vi "Save Selected Area in Image.vi"(6 "Selected Area in Object":T3, 7 "Saved Image File Format":T1, 8 "error in (no error)":errorcluster, 10 "Image Data":T2, 11 "File Path in":path) -> (0 "error out":errorcluster, 3 "File Path out":path)   [LabVIEW 2021]
uses:
  Selected Area in Object.ctl
  <vilib>/picture/picture.llb/imagedata.ctl
  Pictures/Save File Format.ctl
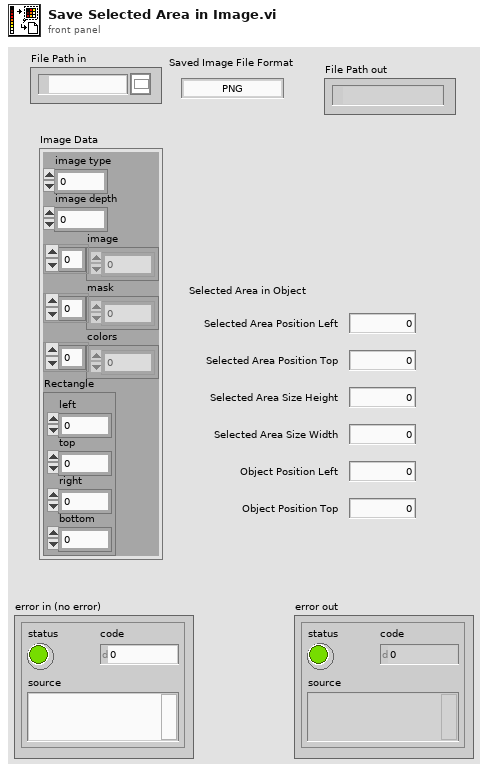
[diagram p1: front panel]
types:
  T1 = typedef "Save File Format.ctl" = enum16{"PNG", "JPEG", "BMP"}
  T2 = typedef "imagedata.ctl" = cluster{"image type":i32, "image depth":i32, "image":u8[], "mask":u8[], "colors":u32[], "Rectangle":cluster{"left":i16, "top":i16, "right":i16, "bottom":i16}}
  T3 = typedef "Selected Area in Object.ctl" = cluster{"Selected Area Position Left":i32, "Selected Area Position Top":i32, "Selected Area Size Height":u32, "Selected Area Size Width":u32, "Object Position Left":i32, "Object Position Top":i32}
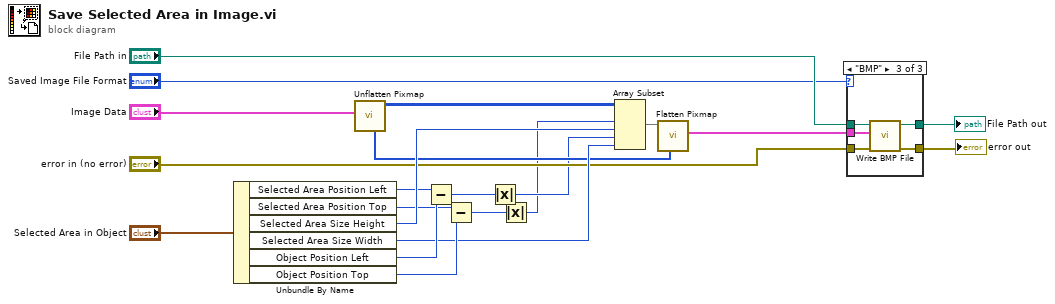
[diagram p0: block diagram]
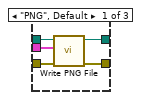
[diagram p2: hidden frame]
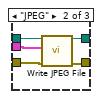
[diagram p3: hidden frame]
diagram:
  n1 = Unbundle By Name("Selected Area in Object") -> ("Selected Area Position Left"=w16:i32, "Selected Area Position Top"=w17:i32, "Selected Area Size Height"=w18:u32, "Selected Area Size Width"=w19:u32, "Object Position Left"=w20:i32, "Object Position Top"=w21:i32)
  n2 = call <vilib>:"Unflatten Pixmap.vi"("image data"="Image Data") -> ("24-bit pixmap"=w6:u32[][], "colors"=w8:u32[])  [unwired: 4 in, 5 out]
  n3 = Subtract(x=w16, y=w20) -> (x-y=w13:i32)
  n4 = Subtract(x=w17, y=w21) -> (x-y=w12:i32)
  n5 = Absolute Value(x=w13) -> (abs(x)=w2:i32)
  n6 = Absolute Value(x=w12) -> (abs(x)=w1:i32)
  n7 = Array Subset(array=w6, index (row)=w1, length (row)=w18, index (col)=w2, length (col)=w19) -> (w7:u32[][])
  n8 = call <vilib>:"Flatten Pixmap.vi"("colors"=w8, "24-bit pixmap"=w7) -> ("image data"=w9:T2)  [unwired: 9 in]
  n9 = case shown="\"BMP\"" "Saved Image File Format" {
    tunnel: "File Path in" -> [w26 w31 w36]
    tunnel: w9 -> [w23 w30 w35]
    tunnel: "error in (no error)" -> [w24 w29 w34]
    tunnel: [w25 w28 w33] -> w11
    tunnel: [w22 w27 w32] -> w14
    frame "PNG", Default {
      n10 = call <vilib>:"Write PNG File.vi"("error in (no error)"=w24, "image data"=w23, "path to PNG file"=w26) -> ("error out"=w25:errorcluster, "path"=w22:path)  [unwired: 7 in]
    }
    frame "JPEG" {
      n11 = call <vilib>:"Write JPEG File.vi"("error in (no error)"=w29, "image data"=w30, "path to JPEG file"=w31) -> ("error out"=w28:errorcluster, "path"=w27:path)  [unwired: 7 in]
    }
    frame "BMP" {
      n12 = call <vilib>:"Write BMP File.vi"("error in (no error)"=w34, "image data"=w35, "path to BMP file"=w36) -> ("error out"=w33:errorcluster, "path"=w32:path)  [unwired: 7 in]
    }
  }
  "File Path out" <- w14
  "error out" <- w11
